vi "ExplorerTree Recursive Files_Folders.vi"(4 "Folder to Exclude":string[](array[string]), 6 "Pattern":string, 8 "error in (no error)":errorcluster, 9 "Continue Recursing on Error? (F)":bool, 11 "Folder Path":path) -> (0 "error out":errorcluster, 1 "Folder Indexes":i32[](array[numeric]), 2 "Folders and Files":path[](array[path]), 3 "dup Folder Path":path)   [LabVIEW 2015]
doc: "List the content of a folder sorted by directories first. The <b>Folder Indexes</b> contain the index locations of the directories in the <b>Folders and Files</b> paths array. All other indexes are files.\n\nCreated By: Ryan Pacini"
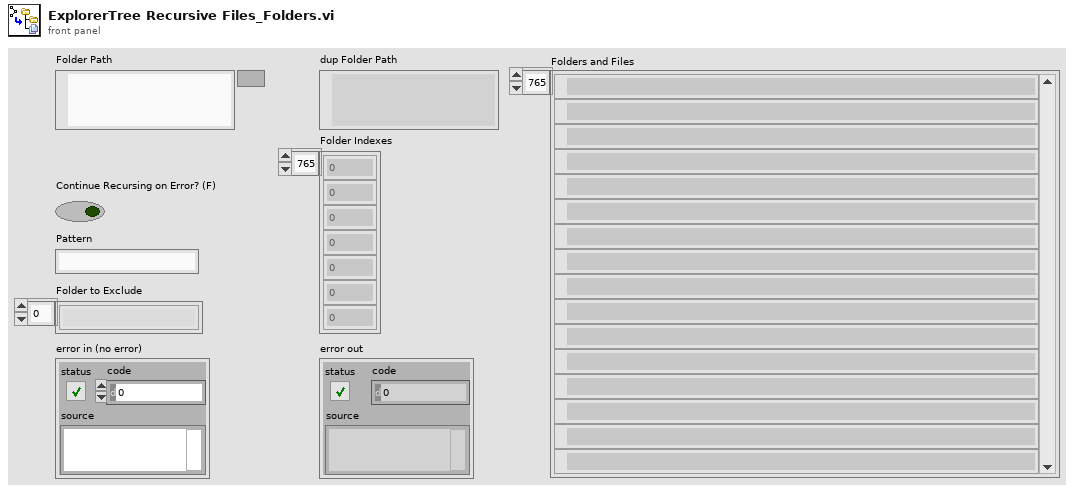
[diagram p1: front panel]
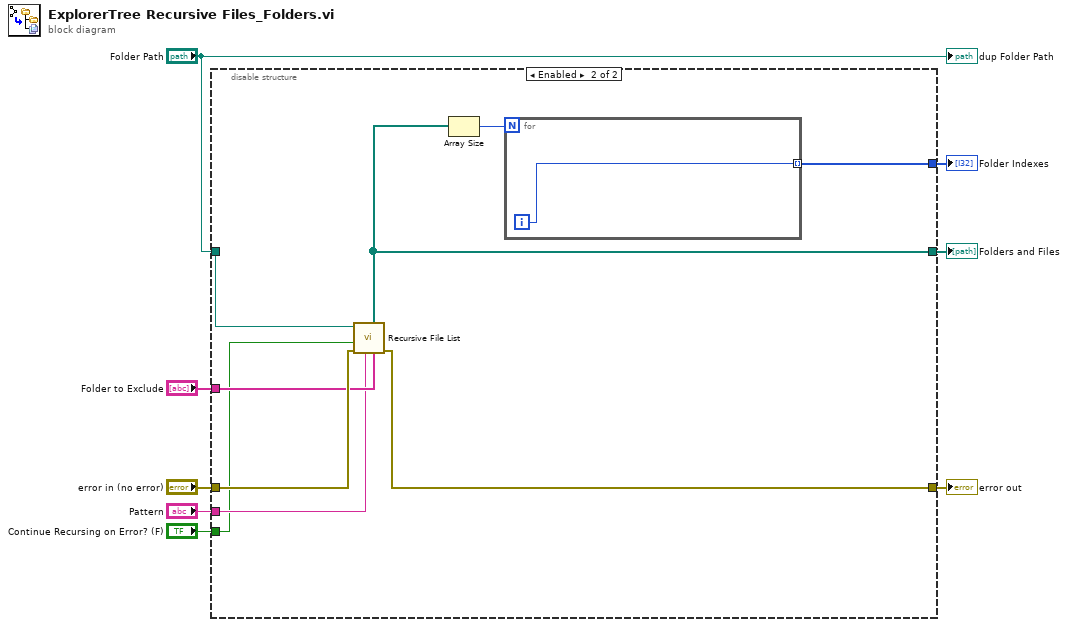
[diagram p0: block diagram]
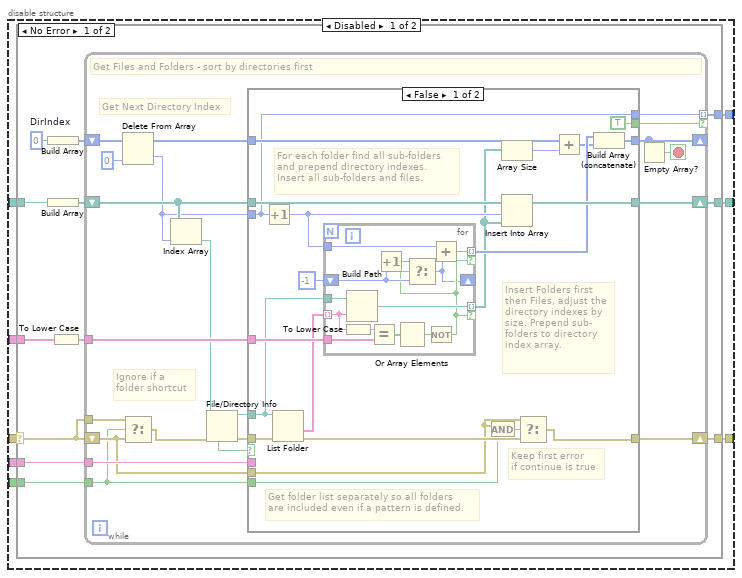
[diagram p2: hidden frame]
diagram:
  n1 = disable-structure shown="Enabled" {
    disable-tunnel: "Folder to Exclude" -> [w16 w94]
    disable-tunnel: [w15 w91] -> w7
    disable-tunnel: "Pattern" -> [w14 w93]
    disable-tunnel: [w13 w89] -> w5
    disable-tunnel: "Folder Path" -> [w12 w96]
    disable-tunnel: "error in (no error)" -> [w11 w95]
    disable-tunnel: "Continue Recursing on Error? (F)" -> [w10 w92]
    disable-tunnel: [w9 w88] -> w1
    frame Disabled {
      n2 = case shown="No Error" w11 {
        selector: w11 -> [w19 w87]
        tunnel: w16 -> [w28 _]
        tunnel: [w26 w87] -> w15
        tunnel: w14 -> [w25 _]
        tunnel: [w21 _] -> w13
        tunnel: w12 -> [w20 _]
        tunnel: w10 -> [w18 _]
        tunnel: [w17 _] -> w9
        frame No Error {
          w23 = 0  # DirIndex
          n3 = Build Array(w23) -> (w22:i32[])
          n4 = Build Array(w20) -> (w24:path[])
          n5 = To Lower Case(string=w28) -> (all lower case string=w27:string[])
          n6 = while {
            tunnel: w27 -> [w45]
            tunnel: w25 -> [w44]
            shift-right: [w43] -> w21
            shift-left: w24 -> [w42]
            shift-right: [w36] -> _
            shift-left: w22 -> [w40]
            shift-right: [w31] -> w26
            shift-left: w19 -> [w33]
            tunnel: w19 -> [w34]
            tunnel: w18 -> [w32]
            tunnel: [w30] -> w17 mode=indexing if=w29
            stop <- w46 stop-if-true
            # "Ignore if a\nfolder shortcut"
            # "Get Next Directory Index"
            # "Get Files and Folders - sort by directories first"
            n7 = Delete From Array(array=w40, index=0) -> (deleted portion=w39:i32, array with subset deleted=w37:i32[])  [unwired: 1 in]
            n8 = Select(t=w34, s=w32, f=w33) -> (s? t:f=w35:errorcluster)
            n9 = Index Array(array=w42, index=w39) -> (element=w41:path)
            n10 = File/Directory Info(path=w41, error in=w35) -> (path out=w48:path, error out=w49:errorcluster, shortcut=w47:bool)  [unwired: 4 out]
            n11 = case shown="False" w47 {
              tunnel: w49 -> [w70 w86]
              tunnel: w48 -> [w67 _]
              tunnel: [w57 w86] -> w31
              tunnel: w45 -> [w69 _]
              tunnel: [w66 w85] -> w43
              tunnel: w44 -> [_ _]
              tunnel: w42 -> [w65 w85]
              tunnel: w39 -> [w53 _]
              tunnel: w37 -> [w60 w84]
              tunnel: [w62 w84] -> w36
              tunnel: w33 -> [w55 _]
              tunnel: w32 -> [w56 _]
              tunnel: [w53 _] -> w30
              tunnel: [TRUE _] -> w29
              frame False {
                # "Keep first error\nif continue is true"
                # "Get folder list separately so all folders \nare included even if a pattern is defined."
                # "For each folder find all sub-folders\nand prepend directory indexes.\nInsert all sub-folders and files."
                # "Insert Folders first\nthen Files, adjust the\ndirectory indexes by\nsize. Prepend sub-\nfolders to directory\nindex array."
                n12 = Increment(x=w53) -> (x+1=w64:i32)
                n13 = List Folder(path=w67, error in=w70) -> (folder names=w68:string[], error out=w58:errorcluster)  [unwired: 2 in, 2 out]
                n14 = for {
                  tunnel: w68 -> [w78] mode=indexing
                  tunnel: w67 -> [w83]
                  tunnel: w69 -> [w81]
                  tunnel: [w77] -> w61 mode=indexing if=w72
                  tunnel: w64 -> [w76]
                  tunnel: [w75] -> w63 mode=indexing if=w72
                  shift-right: [w71] -> _
                  shift-left: -1 -> [w73]
                  # "Exclude Folders"
                  n15 = To Lower Case(string=w78) -> (all lower case string=w82:string)
                  n16 = Build Path(base path=w83, name or relative path=w78) -> (appended path=w77:path)
                  n17 = Equal?(x=w82, y=w81) -> (x = y?=w80:bool[])
                  n18 = Increment(x=w73) -> (x+1=w74:i32)
                  n19 = Or Array Elements(Boolean array=w80) -> (logical OR=w79:bool)
                  n20 = Not(x=w79) -> (.not. x?=w72:bool)
                  n21 = Select(t=w74, s=w72, f=w73) -> (s? t:f=w71:i32)
                  n22 = Add(x=w76, y=w71) -> (x+y=w75:i32)
                }
                n23 = And(x=w55, y=w56) -> (x .and. y?=w54:bool)
                n24 = Array Size(array=w61) -> (size(s)=w50:i32)
                n25 = Insert Into Array(array=w65, index=w64, new element=w61) -> (w66:path[])
                n26 = Select(t=w55, s=w54, f=w58) -> (s? t:f=w57:errorcluster)
                n27 = Add(x=w60, y=w50) -> (x+y=w59:i32[])
                n28 = Build Array (concatenate)(w63, w59) -> (w62:i32[])
              }
              frame True {
                # "Directory is a shortcut, do nothing"
              }
            }
            n29 = Empty Array?(array=w36) -> (empty?=w46:bool)
          }
        }
        frame Error {
        }
      }
    }
    frame Enabled {
      n30 = call <vilib>:"Recursive File List.vi"("Folders to Exclude"=w94, "pattern"=w93, "error in (no error)"=w95, "Continue Recursing on Error? (F)"=w92, "Folder Path"=w96) -> ("error out"=w91:errorcluster, "All Folders"=w89:path[])  [unwired: 2 in, 3 out]
      n31 = Array Size(array=w89) -> (size(s)=w90:i32)
      n32 = for {
        N: w90 -> [_]
        tunnel: [w97] -> w88 mode=indexing
        i -> [w97]
      }
    }
  }
  "error out" <- w7
  "Folders and Files" <- w5
  "Folder Indexes" <- w1
  "dup Folder Path" <- "Folder Path"
